vi "check if brackets Matched.vi"(9 "TYPE":T1(ring), 11 "regular expression":string="[{String:abc;BoolArray:[TRUE,FALSE,TRUE,FALSE]},{String:def;BoolArray:[FALSE,TRUE,FALSE,TRUE]},{String:xyz;BoolArray:[TRUE,TRUE,FALSE,FALSE]}]") -> (0 "Matched?":bool=TRUE, 3 "regular expression (dup)":string="[{String:abc;BoolArray:[TRUE,FALSE,TRUE,FALSE]},{String:def;BoolArray:[FALSE,TRUE,FALSE,TRUE]},{String:xyz;BoolArray:[TRUE,TRUE,FALSE,FALSE]}]")   [LabVIEW 2017, in "API String Arguments Support.lvlib"]
uses:
  API String Arguments Support.lvlib
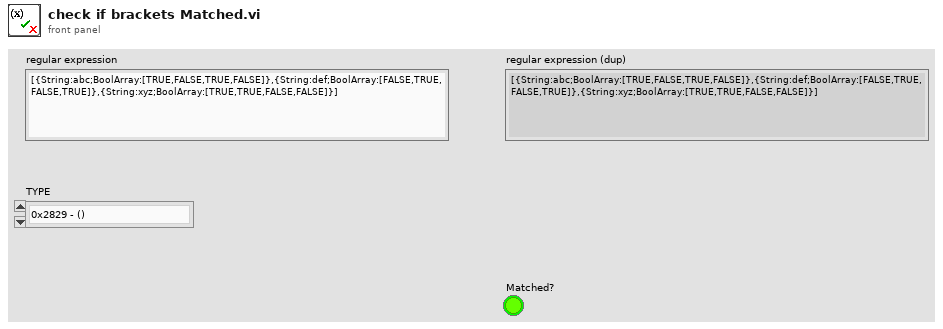
[diagram p1: front panel]
types:
  T1 = enum16{"0x2829 - ()", "0x5B5D - []", "0x7B7D - {}"}
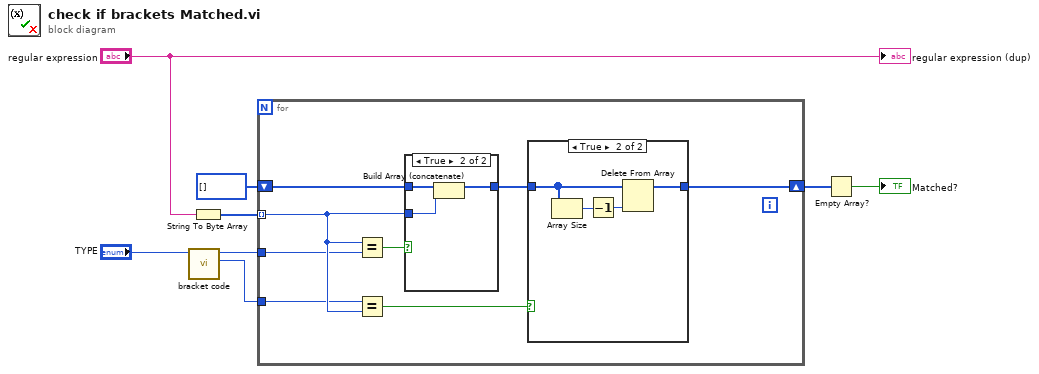
[diagram p0: block diagram]
diagram:
  n1 = call "bracket code.vi"("Enum"="TYPE") -> ("Numeric"=w1:u8, "Numeric 2"=w2:u8)  [unwired: 9 in]
  n2 = String To Byte Array(string="regular expression") -> (unsigned byte array=w7:u8[])
  n3 = for {
    tunnel: w7 -> [w12] mode=indexing
    shift-right: [w11] -> w6
    shift-left: i32[] [] -> [w13]
    tunnel: w2 -> [w10]
    tunnel: w1 -> [w9]
    n4 = Equal?(x=w12, y=w10) -> (x = y?=w16:bool)
    n5 = Equal?(x=w9, y=w12) -> (x = y?=w14:bool)
    n6 = case shown="True" w16 {
      tunnel: w13 -> [w22 w25]
      tunnel: w12 -> [_ w24]
      tunnel: [w22 w23] -> w15
      frame False {
      }
      frame True {
        n7 = Build Array (concatenate)(w25, w24) -> (w23:i32[])
      }
    }
    n8 = case shown="True" w14 {
      tunnel: w15 -> [w17 w20]
      tunnel: [w17 w18] -> w11
      frame False {
      }
      frame True {
        n9 = Array Size(array=w20) -> (size(s)=w21:i32)
        n10 = Decrement(x=w21) -> (x-1=w19:i32)
        n11 = Delete From Array(array=w20, index=w19) -> (array with subset deleted=w18:i32[])  [unwired: 1 in, 1 out]
      }
    }
  }
  n12 = Empty Array?(array=w6) -> (empty?=→"Matched?":bool)
  "regular expression (dup)" <- "regular expression"
